vi "USRP Throughput Streaming - To Disk (Host).vi"() -> ()   [LabVIEW 2016]
doc: "Example Description:\nAcquires data at the specified rate from a RIO device and writes the data to disk using TDMS asynchronous writes instead of the built-in LabVIEW file I/O.\n\nAsynchronous writes provide for the best possible performance, since the HDD controller can spend more time transferring data than is possible with synchronous blocking writes. Furthermore, since TDMS effectively queues up the data from multiple writes for us, queues on the LabVEIW diagram are no longer necessary, simplifying the application by removing the queue and the separate read and write loops.\n\nVI Configuration:\nThis example uses the PXI-7966R as the FPGA target by default. To use this VI with another FPGA target, use the following steps to configure the host VI to use a VI configured for your FPGA target:\n\n1. On the block diagram, right-click the Open FPGA VI Reference (PXI-7966R) VI and select Configure Open FPGA VI Reference.\n2. Browse for a new target by clicking the Browse Project button in the Open VI section.\n3. Select the VI under the target that matches your device. Click OK to select this VI.\n4. Click OK to exit the dialog box and to apply the new selection to the FPGA VI.\n\nRunning the VI:\n1. Select a RIO Resource that corresponds to the FPGA device configured above.\n2. Select a source TDMS file that you will be streaming data to.\n3. Configure the Acquisition Size, Requested host Buffer Depth, Read Size, MAX TDMS Asynchronous Writes, and Requested (M) controls on the Host VI Front Panel.\n4. Click the run arrow to run the VI.\n5. Observe the Status of the Host Buffer as well as the Input DMA FIFO.\n6. Observe the achieved Streaming Throughput.\n7. Click Stop on the Front Panel to stop the example\n\n\nExecution Steps:\nRefer to the block diagram of the Host VI for each example to view the execution steps for that specific example."
uses:
  <vilib>/rvi/interface/nirviOpenFPGA/nirviOpenFPGA.xnode
  <vilib>/rvi/interface/nirviMethod/nirviMethod.xnode
  <vilib>/rvi/interface/nirviReadWriteControl/nirviReadWriteControl.xnode
  <vilib>/rvi/interface/Simulation/niFpgaSimulationCallBeginRW.vi
  <vilib>/rvi/errors/niLvFpgaAdjustHostInterfaceError.vi
  <vilib>/rvi/interface/nirviCloseFPGA/nirviCloseFPGA.xnode
  <vilib>/rvi/errors/niLvFpgaMergeErrorWithErrorCode.vi
  NiFpgaLv.dll
  <vilib>/Utility/error.llb/Error Cluster From Error Code.vi
  <vilib>/FPGAPlugInAG/Dynamic/niLvFpga_Run_Dynamic.vi
  FPGA Bitfiles/USRP-RIO-Streami_FlexRIOHighThrou_USRPThroughputSt_y+O3+0ZwI2I.lvbitx
  <vilib>/FPGAPlugInAG/USRP 294xR; 295xR 200 MSps/niLvFpga_Open_USRP 294xR; 295xR 200 MSps.vi
  <vilib>/rvi/interface/common/dynamic/niFpgaDynamicAddResources.vi
  <vilib>/FPGAPlugInAG/Dynamic/niLvFpga_ConfigureFifo_Dynamic.vi
  <vilib>/FPGAPlugInAG/Dynamic/niLvFpga_StartFifo_Dynamic.vi
  <vilib>/FPGAPlugInAG/Dynamic/niLvFpga_AcquireReadRegionFifo_Dynamic.vi
  <vilib>/FPGAPlugInAG/Dynamic/niLvFpga_Close_Dynamic.vi
  <vilib>/userdefined/High Color/nirio_resource_hc.ctl
panel:
  out "Max Pending TDMS Writes":u32 caption="Max Pending"
  out "Pending TDMS Writes":u32 caption="Pending"
  in  "Max TMDS Asynchronous Writes":u32=8
  in  "file path":path=path "Select a destination TDMS file"
  out "Actual Acquisition Size (samples)":u64 caption="actual acquisition size (samples)"
  out "Host Buffer Depth (samples)":u32
  out "error out":errorcluster
  in  "Stop":bool
  out "input.Ever Timed Out?":bool caption="Overflow"
  in  "input.Reset":bool
  out "Max Throughput":u16 caption="Maximum (M)"
  in  "Requested Throughput":u16=1000 caption="Requested (M)" step=5
  in  "Requested Host Buffer Depth (samples)":u32=67108864 step=1048576
  in  "Read Size (samples)":u32=4194304 step=1048576
  out "Samples Acquired":u64(slide) caption="Acquisition Progress" scale=0.0..1000000000.0 scale format="%#.1p"
  out "Stop...":bool
  out "Host Buffer Status":cluster{u32, u32, u32}(slide) scale=0.0..67108864.0 scale format="%#.1p"
  out "input.Throughput (B/s)":dbl caption="Actual" format="%#.1p"
  out "input.FPGA FIFO Status":cluster{u32, u32}(slide) caption="FIFO Status" scale=0.0..65535.0 scale format="%#.1p"
  in  "Acquisition Size (samples)":u64=1000000000 format="%#.3p"
  in  "resource name":T1="Select RIO resource"
  # "Configuration"
  # "Host"
  # "TDMS Writes"
  # "Input FPGA"
  # "Throughput (B/s)"
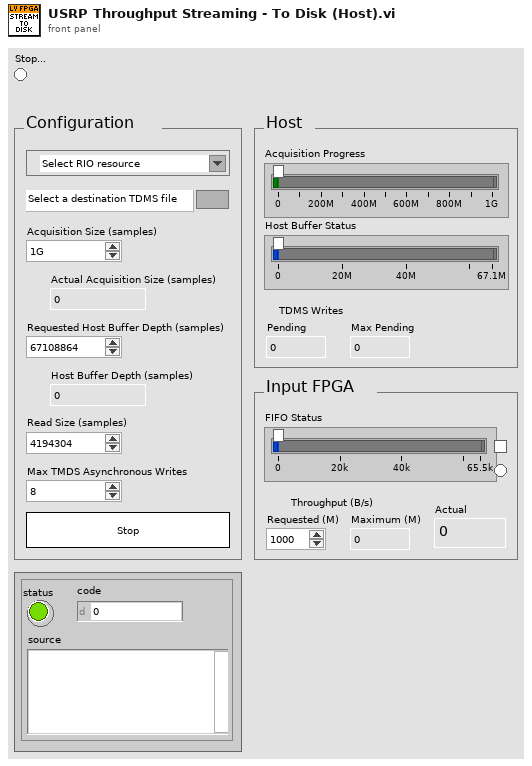
[diagram p1: front panel]
types:
  T1 = typedef "nirio_resource_hc.ctl" = tag
  T2 = enum16{"open", "open or create", "create or replace", "create", "open (read-only)"}
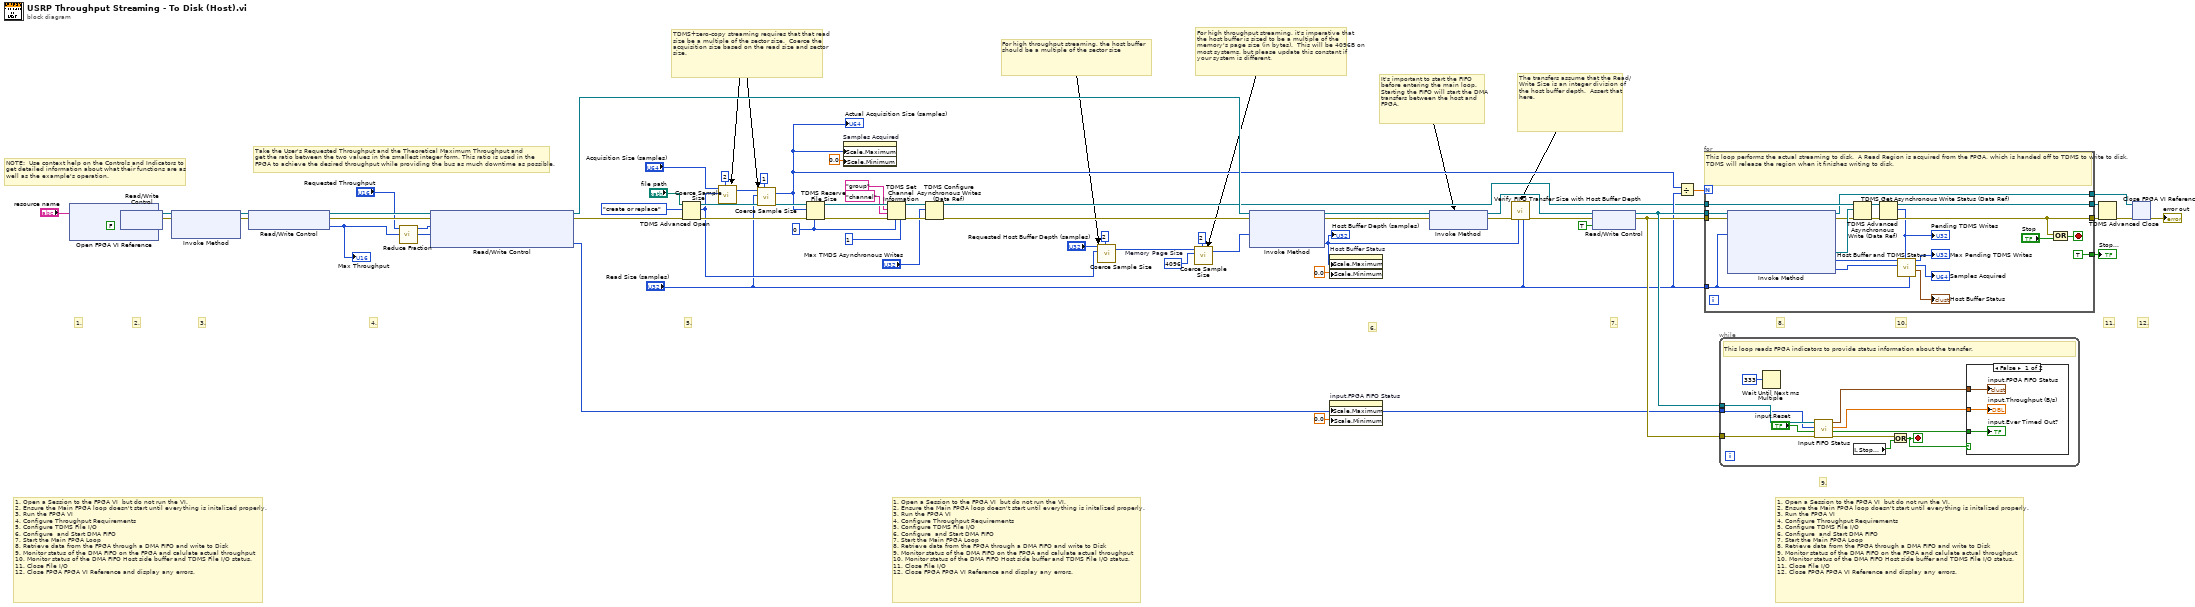
[diagram p0: block diagram]
diagram:
  w26 = u64 4096  # Memory Page Size
  w42 = i16 0 ("data type")
  # "Take the User's Requested Throughput and the Theoretical Maximum Throughput and\nget the ratio between the two values in the smallest integer form. This ratio is used in the \nFPGA to achieve the desired throughput while providing the bus as much downtime as possible."
  # "1. Open a Session to the FPGA VI  but do not run the VI.\n2. Ensure the Main FPGA loop doesn't start until everything is initalized properly. \n3. Run the FPGA VI\n4. Configure Throughput Requirements\n5. Configure TDMS File I/O\n6. Configure  and Start DMA FIFO\n7. Start the Main FPGA Loop\n8. Retrieve data from the FPGA through a DMA FIFO and write to Disk\n9. Monitor status of the DMA FIFO on the FPGA and calulate actual throughput\n10. Monitor status of the DMA FIFO Host side buffer and TDMS File I/O status.\n11. Close File I/O\n12. Close FPGA FPGA VI Reference and display any errors."
  # "1. Open a Session to the FPGA VI  but do not run the VI.\n2. Ensure the Main FPGA loop doesn't start until everything is initalized properly. \n3. Run the FPGA VI\n4. Configure Throughput Requirements\n5. Configure TDMS File I/O\n6. Configure  and Start DMA FIFO\n7. Start the Main FPGA Loop\n8. Retrieve data from the FPGA through a DMA FIFO and write to Disk\n9. Monitor status of the DMA FIFO on the FPGA and calulate actual throughput\n10. Monitor status of the DMA FIFO Host side buffer and TDMS File I/O status.\n11. Close File I/O\n12. Close FPGA FPGA VI Reference and display any errors."
  # "9."
  # "10."
  # "12."
  # "11."
  # "8."
  # "7."
  # "6."
  # "5."
  # "4."
  # "3."
  # "2."
  # "1. Open a Session to the FPGA VI  but do not run the VI.\n2. Ensure the Main FPGA loop doesn't start until everything is initalized properly. \n3. Run the FPGA VI\n4. Configure Throughput Requirements\n5. Configure TDMS File I/O\n6. Configure  and Start DMA FIFO\n7. Start the Main FPGA Loop\n8. Retrieve data from the FPGA through a DMA FIFO and write to Disk\n9. Monitor status of the DMA FIFO on the FPGA and calulate actual throughput\n10. Monitor status of the DMA FIFO Host side buffer and TDMS File I/O status.\n11. Close File I/O\n12. Close FPGA FPGA VI Reference and display any errors."
  # "1."
  # "NOTE:  Use context help on the Controls and Indicators to \nget detailed information about what their functions are as\nwell as the example's operation."
  # "The transfers assume that the Read/Write Size is an integer division of the host buffer depth.  Assert that here."
  # "It's important to start the FIFO before entering the main loop.  Starting the FIFO will start the DMA transfers between the host and FPGA."
  # "TDMS+zero-copy streaming requires that that read size be a multiple of the sector size.  Coerce the acquisition size based on the read size and sector size."
  # "For high throughput streaming, it's imperative that the host buffer is sized to be a multiple of the memory's page size (in bytes).  This will be 4096B on most systems, but please update this constant if your system is different."
  # "For high throughput streaming, the host buffer should be a multiple of the sector size"
  n1 = xnode "Open FPGA VI Reference"("resource name"="resource name") -> ("FPGA VI Reference Out"=w53:refnum<k20>, "error out"=w58:errorcluster)  [unwired: 1 in]
  n2 = xnode "Read/Write Control"("FPGA VI Reference In"=w53, "error in"=w58, "input.Start"=FALSE) -> ("FPGA VI Reference Out"=w54:refnum<k20>, "error out"=w56:errorcluster)
  n3 = xnode "Invoke Method"("FPGA VI Reference In"=w54, "error in"=w56) -> ("FPGA VI Reference Out"=w10:refnum<k20>, "error out"=w9:errorcluster)  [unwired: 1 in]
  n4 = xnode "Read/Write Control"("FPGA VI Reference In"=w10, "error in"=w9) -> ("FPGA VI Reference Out"=w8:refnum<k20>, "error out"=w7:errorcluster, "input.Max Throughput"=w5:u16)
  "Max Throughput" <- w5
  n5 = call "Reduce Fraction.vi"("denominator"=w5, "numerator"="Requested Throughput") -> ("reduced denominator"=w4:u16, "reduced numerator"=w3:u16)  [unwired: 2 in]
  n6 = xnode "Read/Write Control"("FPGA VI Reference In"=w8, "error in"=w7, "input.Requested Throughput"=w3, "input.Requested Throughput Denominator"=w4) -> ("FPGA VI Reference Out"=w15:refnum<k20>, "error out"=w38:errorcluster, "input.FIFO Size"=w49:u32)
  n7 = TDMS Advanced Open(8:w38, 10:T2."create or replace" ("operation (0:open)"), 11:"file path") -> (0:w37:errorcluster, 2:w29:u32, 3:w48:refnum<k34>)  [unwired: 2 in]
  n8 = call "Coerce Sample Size.vi"("Bytes Per Sample (B)"=u64 2, "Coerce To (B)"=w29, "Size (samples)"="Acquisition Size (samples)") -> ("Coerced Size (samples)"=w35:u64)  [unwired: 4 in]
  n9 = call "Coerce Sample Size.vi"("Bytes Per Sample (B)"=u64 1, "Coerce To (B)"="Read Size (samples)", "Size (samples)"=w35) -> ("Coerced Size (samples)"=w2:u64)  [unwired: 4 in]
  "Actual Acquisition Size (samples)" <- w2
  n10 = TDMS Reserve File Size(6:w42, 8:w37, 10:w2, 11:w48) -> (0:w43:errorcluster, 3:w47:refnum<k34>)  [unwired: 1 in]
  n11 = property on="Samples Acquired" class="Slide (strict)"("Scale.Maximum"=w2, "Scale.Minimum"=0.0 ("Scale.Range:Minimum")) -> ()  [unwired: 2 in, 2 out]
  n12 = TDMS Set Channel Information(4:u32 1 ("samples per channel"), 6:w42, 8:w43, 9:"channel" ("group name (Untitled)"), 10:"group" ("group name (Untitled)"), 11:w47) -> (0:w36:errorcluster, 3:w46:refnum<k34>)  [unwired: 1 in]
  n13 = TDMS Configure Asynchronous Writes (Data Ref)(8:w36, 10:"Max TMDS Asynchronous Writes", 11:w46) -> (0:w22:errorcluster, 3:w14:refnum<k34>)  [unwired: 1 in]
  n14 = call "Coerce Sample Size.vi"("Bytes Per Sample (B)"=u64 2, "Coerce To (B)"=w29, "Size (samples)"="Requested Host Buffer Depth (samples)") -> ("Coerced Size (samples)"=w25:u64)  [unwired: 4 in]
  n15 = call "Coerce Sample Size.vi"("Bytes Per Sample (B)"=u64 2, "Coerce To (B)"=w26, "Size (samples)"=w25) -> ("Coerced Size (samples)"=w24:u64)  [unwired: 4 in]
  n16 = xnode "Invoke Method"("FPGA VI Reference In"=w15, "error in"=w22, "Requested Depth"=w24) -> ("FPGA VI Reference Out"=w20:refnum<k20>, "error out"=w21:errorcluster, "Actual Depth"=w1:u32)
  "Host Buffer Depth (samples)" <- w1
  n17 = property on="Host Buffer Status" class="Slide (strict)"("Scale.Maximum"=w1, "Scale.Minimum"=0.0 ("Scale.Range:Minimum")) -> ()  [unwired: 2 in, 2 out]
  n18 = property on="input.FPGA FIFO Status" class="Slide (strict)"("Scale.Maximum"=w49, "Scale.Minimum"=0.0 ("Scale.Range:Minimum")) -> ()  [unwired: 2 in, 2 out]
  n19 = xnode "Invoke Method"("FPGA VI Reference In"=w20, "error in"=w21) -> ("FPGA VI Reference Out"=w17:refnum<k20>, "error out"=w19:errorcluster)
  n20 = call "Verify FIFO Transfer Size with Host Buffer Depth.vi"("Read/Write Size (samples)"="Read Size (samples)", "Host Buffer Depth (samples)"=w1, "error in"=w19) -> ("error out"=w16:errorcluster)  [unwired: 8 in]
  n21 = xnode "Read/Write Control"("FPGA VI Reference In"=w17, "error in"=w16, "input.Start"=TRUE ("Start")) -> ("FPGA VI Reference Out"=w52:refnum<k20>, "error out"=w51:errorcluster)
  n22 = Divide(x=w2, y="Read Size (samples)") -> (x/y=w11:dbl)
  n23 = for {
    N: w11 -> [_]
    tunnel: w52 -> [w84]
    tunnel: w14 -> [w83]
    tunnel: w51 -> [w82]
    tunnel: [w75] -> w63
    tunnel: "Read Size (samples)" -> [w65]
    tunnel: [TRUE] -> w59
    tunnel: [w74] -> w13
    tunnel: [w67] -> w12
    stop <- w78 stop-if-true
    # "This loop performs the actual streaming to disk.  A Read Region is acquired from the FPGA, which is handed off to TDMS to write to disk.  TDMS will release the region when it finishes writing to disk."
    n24 = xnode "Invoke Method"("FPGA VI Reference In"=w84, "error in"=w82, "Number of Elements"=w65) -> ("FPGA VI Reference Out"=w67:refnum<k20>, "error out"=w79:errorcluster, "Read Region Reference"=w80:refnum<data-value>, "Elements In Region"=w73:u32, "Elements Remaining"=w72:u32)  [unwired: 1 in]
    n25 = TDMS Advanced Asynchronous Write (Data Ref)(8:w79, 10:w80, 11:w83) -> (0:w77:errorcluster, 3:w76:refnum<k34>)  [unwired: 1 in]
    n26 = TDMS Get Asynchronous Write Status (Data Ref)(8:w77, 11:w76) -> (0:w75:errorcluster, 2:w71:u32, 3:w74:refnum<k34>)
    "Pending TDMS Writes" <- w71
    n27 = call "Host Buffer and TDMS Status.vi"("Read/Write Size (samples)"=w65, "Number of Pending Reads/Writes"=w71, "Elements Remaining"=w72, "Elements In Region"=w73) -> ("Host Buffer Status"=→"Host Buffer Status":cluster{u32, u32, u32}, "Samples Transferred"=→"Samples Acquired":u64, "Running Max of TDMS Reads/Writes"=→"Max Pending TDMS Writes":u32)  [unwired: 5 in]
    n28 = Compound Arithmetic op=OR(w75, "Stop") -> (w78:bool)
  }
  "Stop..." <- w59
  n29 = while {
    tunnel: w52 -> [w95]
    tunnel: w51 -> [w93]
    tunnel: w49 -> [w88]
    stop <- w85 stop-if-true
    # "This loop reads FPGA indicators to provide status information about the transfer."
    n30 = Wait Until Next ms Multiple(millisecond multiple=u32 333) -> ()  [unwired: 1 out]
    n31 = call "Input FIFO Status.vi"("error in"=w93, "input.Reset"="input.Reset", "input.FIFO Size"=w88, "FPGA VI Reference"=w95) -> ("error out"=w87:errorcluster, "input.Ever Timed Out?"=w90:bool, "input.Throughput (B/s)"=w91:dbl, "input.FPGA FIFO Status"=w92:cluster{u32, u32})  [unwired: 3 in]
    n32 = local read "Stop..."() -> (w86:bool)
    n33 = Or(x=w87, y=w86) -> (x .or. y?=w85:bool)
    n34 = case shown="False" w85 {
      tunnel: w92 -> [w98 _]
      tunnel: w91 -> [w97 _]
      tunnel: w90 -> [w96 _]
      frame False {
        "input.Throughput (B/s)" <- w97
        "input.Ever Timed Out?" <- w96
        "input.FPGA FIFO Status" <- w98
      }
      frame True {
      }
    }
  }
  n35 = TDMS Advanced Close(8:w63, 11:w13) -> (0:w62:errorcluster)  [unwired: 2 in, 1 out]
  n36 = xnode "Close FPGA VI Reference"("FPGA VI Reference In"=w12, "error in"=w62) -> ("error out"=→"error out":errorcluster)
